vi "CLItest.vi"() -> ()   [LabVIEW 2012]
panel:
  in  "Write?":bool
  out "String":string
  in  "Hatches":T1(array[cluster])=[{"Start"={"X"=0.0, "Y"=0.0}, "End"={"X"=2.0, "Y"=0.0}}, {"Start"={"X"=0.0, "Y"=1.0}, "End"={"X"=2.0, "Y"=1.0}}, {"Start"={"X"=0.0, "Y"=2.0}, "End"={"X"=2.0, "Y"=2.0}}]
  in  "PolyLine":cluster{"X":dbl, "Y":dbl}[](array[cluster])=[{"X"=0.0, "Y"=0.0}, {"X"=5.0, "Y"=6.0}, {"X"=2.0, "Y"=4.0}, {"X"=5.0, "Y"=2.0}, {"X"=3.0, "Y"=4.0}]
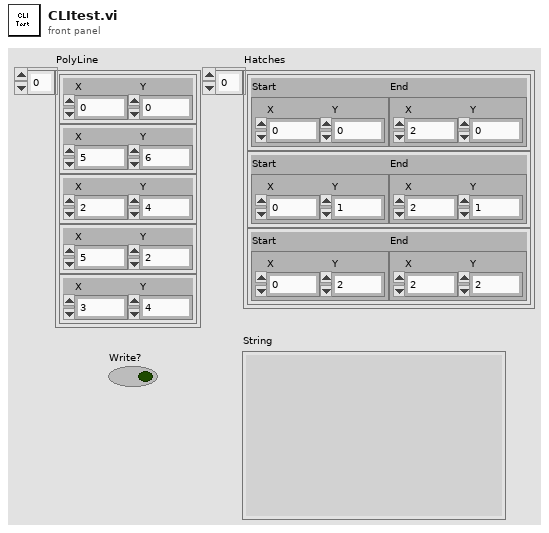
[diagram p1: front panel]
types:
  T1 = cluster{"Start":cluster{"X":dbl, "Y":dbl}, "End":cluster{"X":dbl, "Y":dbl}}[]
  T2 = enum16{"HeaderStart", "HeaderEnd", "Binary", "Units"}
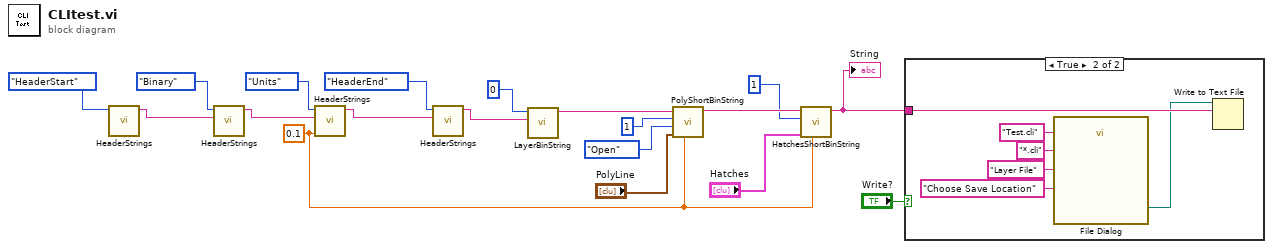
[diagram p0: block diagram]
diagram:
  w6 = 0.1 ("Units")
  n1 = call "HeaderStrings.vi"("Type"=T2."HeaderStart") -> ("ASCIIstringOut"=w18:string)  [unwired: 10 in]
  n2 = call "HeaderStrings.vi"("ASCIIstringIn"=w18, "Type"=T2."Binary") -> ("ASCIIstringOut"=w16:string)  [unwired: 9 in]
  n3 = call "HeaderStrings.vi"("Units"=w6, "ASCIIstringIn"=w16, "Type"=T2."Units") -> ("ASCIIstringOut"=w14:string)  [unwired: 8 in]
  n4 = call "HeaderStrings.vi"("ASCIIstringIn"=w14, "Type"=T2."HeaderEnd") -> ("ASCIIstringOut"=w3:string)  [unwired: 9 in]
  n5 = call "LayerBinString.vi"("BinStringIn"=w3, "Layer"=u16 0) -> ("BinStringOut"=w2:string)  [unwired: 9 in]
  n6 = call "PolyShortBinString.vi"("Units"=w6, "PolyLine"="PolyLine", "Dir"=enum16{"CW", "CCW", "Open"}."Open", "ID"=u16 1, "BinStirngIn"=w2) -> ("String"=w9:string)  [unwired: 6 in]
  n7 = call "HatchesShortBinString.vi"("Units"=w6, "Hatches"="Hatches", "ID"=u16 1, "BinStirngIn"=w9) -> ("String"=w5:string)  [unwired: 7 in]
  "String" <- w5
  n8 = case shown="True" "Write?" {
    tunnel: w5 -> [_ w25]
    frame False {
    }
    frame True {
      n9 = call "File Dialog"("prompt"="Choose Save Location", "default name"="Test.cli", "pattern (all files)"="*.cli", "pattern label"="Layer File") -> ("selected path"=w24:path)  [unwired: 8 in, 3 out]
      n10 = Write to Text File(file (use dialog)=w24, text=w25) -> ()  [unwired: 2 in, 3 out]
    }
  }
